vi "结构相似性设置.vi"(11 "图像输入":T1) -> (0 "error out":errorcluster, 3 "结构相似性图像":T1(plugin-control))   [LabVIEW 2018]
uses:
  <vilib>/vision/Image Controls.llb/IMAQ Image.ctl
  <vilib>/vision/NI_Vision_Development_Module.lvlib
panel:
  out "error out":errorcluster
  in  "细分":i32=8
  in  "对比图像路径":path=path "C:/Users/Lenovo/Desktop/vision/img/1.png"
  in  "关闭":bool
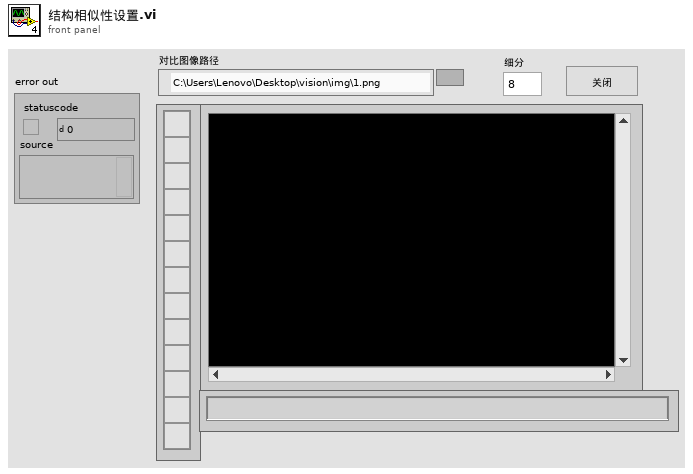
[diagram p1: front panel]
types:
  T1 = typedef "IMAQ Image.ctl" = refnum<image>
  T2 = typedef "Image Type" = u32
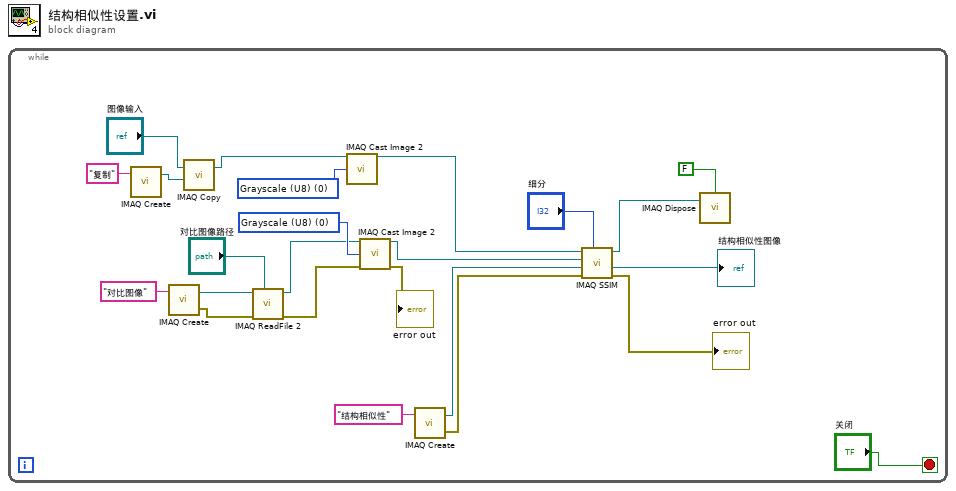
[diagram p0: block diagram]
diagram:
  n1 = while {
    stop <- "关闭" stop-if-true
    w9 = T2 0 items=["Grayscale (U8)", "Grayscale (I16)", "Grayscale (SGL)", "Complex (CSG)", "RGB (U32)", "HSL (U32)", "RGB (U64)", "Grayscale (U16)"] ("Image Type")
    w13 = T2 0 items=["Grayscale (U8)", "Grayscale (I16)", "Grayscale (SGL)", "Complex (CSG)", "RGB (U32)", "HSL (U32)", "RGB (U64)", "Grayscale (U16)"] ("Image Type")
    n2 = call "IMAQ Create"("Image Name"="复制") -> ("New Image"=w6:T1)  [unwired: 4 in, 1 out]
    n3 = call "IMAQ Create"("Image Name"="对比图像") -> ("New Image"=w20:T1, "error out"=w22:errorcluster)  [unwired: 4 in]
    n4 = call "IMAQ Copy"("Image Dst"=w6, "Image Src"="图像输入") -> ("Image Dst Out"=w4:T1)  [unwired: 4 in, 1 out]
    n5 = call "IMAQ ReadFile 2"("File Path"="对比图像路径", "error in (no error)"=w22, "Image"=w20) -> ("error out"=w11:errorcluster, "Image Out"=w12:T1)  [unwired: 4 in, 3 out]
    n6 = call "IMAQ Cast Image 2"("Image Src"=w4, "Image Type"=w9) -> ("Image Dst Out"=w8:T1)  [unwired: 12 in, 1 out]
    n7 = call "IMAQ Cast Image 2"("Image Src"=w12, "Image Type"=w13, "error in (no error)"=w11) -> ("Image Dst Out"=w10:T1, "error out"=→"error out":errorcluster)  [unwired: 11 in]
    n8 = call "IMAQ Create"("Image Name"="结构相似性") -> ("New Image"=w18:T1, "error out"=w17:errorcluster)  [unwired: 4 in]
    n9 = call-poly "IMAQ SSIM"("Window Size"="细分", "error in (no error)"=w17, "SSIM Image In"=w18, "Reference Image"=w10, "Test Image"=w8) -> ("error out"=→"error out":errorcluster, "SSIM Image Out"=→"结构相似性图像":T1, "Test Image Out (dup)"=w2:T1)  [unwired: 2 in, 2 out]
    n10 = call "IMAQ Dispose"("All Images? (No)"=FALSE, "Image"=w2) -> ()  [unwired: 4 in, 1 out]
  }
